vi "Get CD Engine Event Ref.vi"(11 "Assembler in":refnum<class "Assembler.lvclass">) -> (2 "Get Engine Event Ref":T1, 3 "Assembler out":refnum<class "Assembler.lvclass">)   [LabVIEW 2019, in "TimingDRV Engine.lvlib" / "Assembler.lvclass"]
uses:
  Assembler.lvclass
  <vilib>/NI VeriStand/Custom Device API/Custom Device Engine Event Ref.ctl
  Assembler.lvclass/Assembler.ctl
  <vilib>/NI VeriStand/Custom Device API/Custom Device API.lvlib
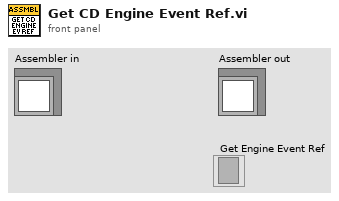
[diagram p1: front panel]
types:
  T1 = typedef "Custom Device API.lvlib/Custom Device Engine Event Ref.ctl" = refnum<event-registration>
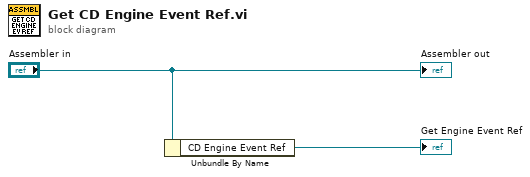
[diagram p0: block diagram]
diagram:
  n1 = Unbundle By Name("Assembler in") -> ("CD Engine Event Ref"=→"Get Engine Event Ref":T1)
  "Assembler out" <- "Assembler in"
